vi "Set Absolute Date Time.vi"(0 "VISA resource name":refnum<visa-resource-name>, 1 "Hour":i32 min=0 max=23 step=1, 5 "Year":i32=1970 min=1970 step=1, 7 "Month":i32=1 min=1 max=12 step=1, 9 "Day":i32=1 min=1 max=31 step=1, 11 "error in (no error)":errorcluster, 12 "Minute":i32 min=0 max=59 step=1) -> (4 "VISA resource name out":refnum<visa-resource-name>, 15 "error out":errorcluster)   [LabVIEW 2018, in "Keithley DMM7512.lvlib"]
doc: "This sets the System Time Year, Month, Day, Hour, Minute, Second."
uses:
  <instrlib>/Keithley DMM7512/Keithley DMM7512.lvlib
panel:
  in  "Second":i32 min=0 max=59 step=1
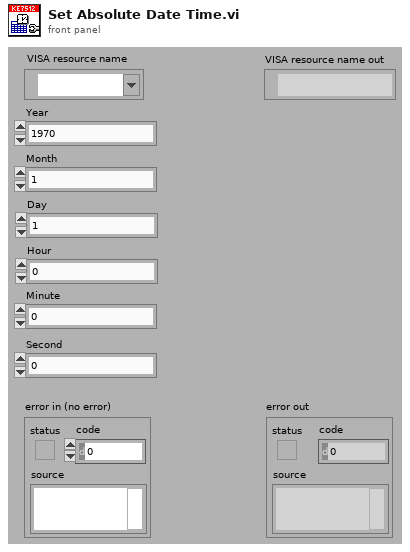
[diagram p1: front panel]
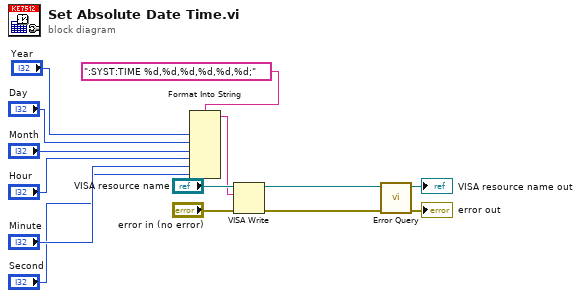
[diagram p0: block diagram]
diagram:
  n1 = Format Into String(format string=":SYST:TIME %d,%d,%d,%d,%d,%d;", "Year", "Day", "Month", "Hour", "Minute", "Second") -> (resulting string=w3:string)  [unwired: 2 in, 1 out]
  n2 = VISA Write(VISA resource name="VISA resource name", write buffer=w3, error in (no error)="error in (no error)") -> (VISA resource name out=w2:refnum<visa-resource-name>, error out=w1:errorcluster)  [unwired: 1 out]
  n3 = call <instrlib>:"Error Query.vi"("error in (no error)"=w1, "VISA resource name"=w2) -> ("error out"=→"error out":errorcluster, "VISA resource name out"=→"VISA resource name out":refnum<visa-resource-name>)  [unwired: 8 out]
